vi "J1939 - SPN Indicator.vi"() -> ()   [LabVIEW 2023, in "J1939 Workspace Object.lvlib"]
doc: "Sample numeric display item."
uses:
  J1939 Workspace Object.lvlib
  <vilib>/NI VeriStand/Display Template Support/DisplayTemplateSupport.llb/cluster_Screen Item Settings.ctl
  <vilib>/NI VeriStand/Display Template Support/DisplayTemplateSupport.llb/cluster_Graph Scale Settings.ctl
  <vilib>/NI VeriStand/Display Template Support/DisplayTemplateSupport.llb/cluster_Graph Plot Settings.ctl
  NationalInstruments.VeriStand.SystemStorage
  Addon/Addon Shared/Types/SPN Properties.ctl
  <vilib>/NI VeriStand/Display Template Support/DisplayTemplateSupport.llb/enum_Display Template Handler Minimal To Workspace.ctl
  <vilib>/NI VeriStand/Display Template Support/DisplayTemplateSupport.llb/enum_Display Template Handler Minimal To Widget Msg.ctl
  <vilib>/NI VeriStand/Execution/Workspace/NI VeriStand - Get Single Channel Value.vi
  <vilib>/NI VeriStand/Display Template Support/DisplayTemplateSupport.llb/sub_Display Template Handler Custom.vi
  <vilib>/NI VeriStand/Execution/Workspace/NI_VS Workspace ExecutionAPI.lvlib
  Workspace Shared/J1939 Workspace Shared.lvlib
  Addon/Addon Shared/J1939 Addon Shared.lvlib
panel:
  out "Scale Info":T1
  in  "NIVS.System Definition Root":refnum<k24>
  out "Raw":u64 format="%.0x"
  out "MSB":u8 format="%.0x"
  in  "Item.Data":T2
  out "Numeric":dbl format="%.2f"
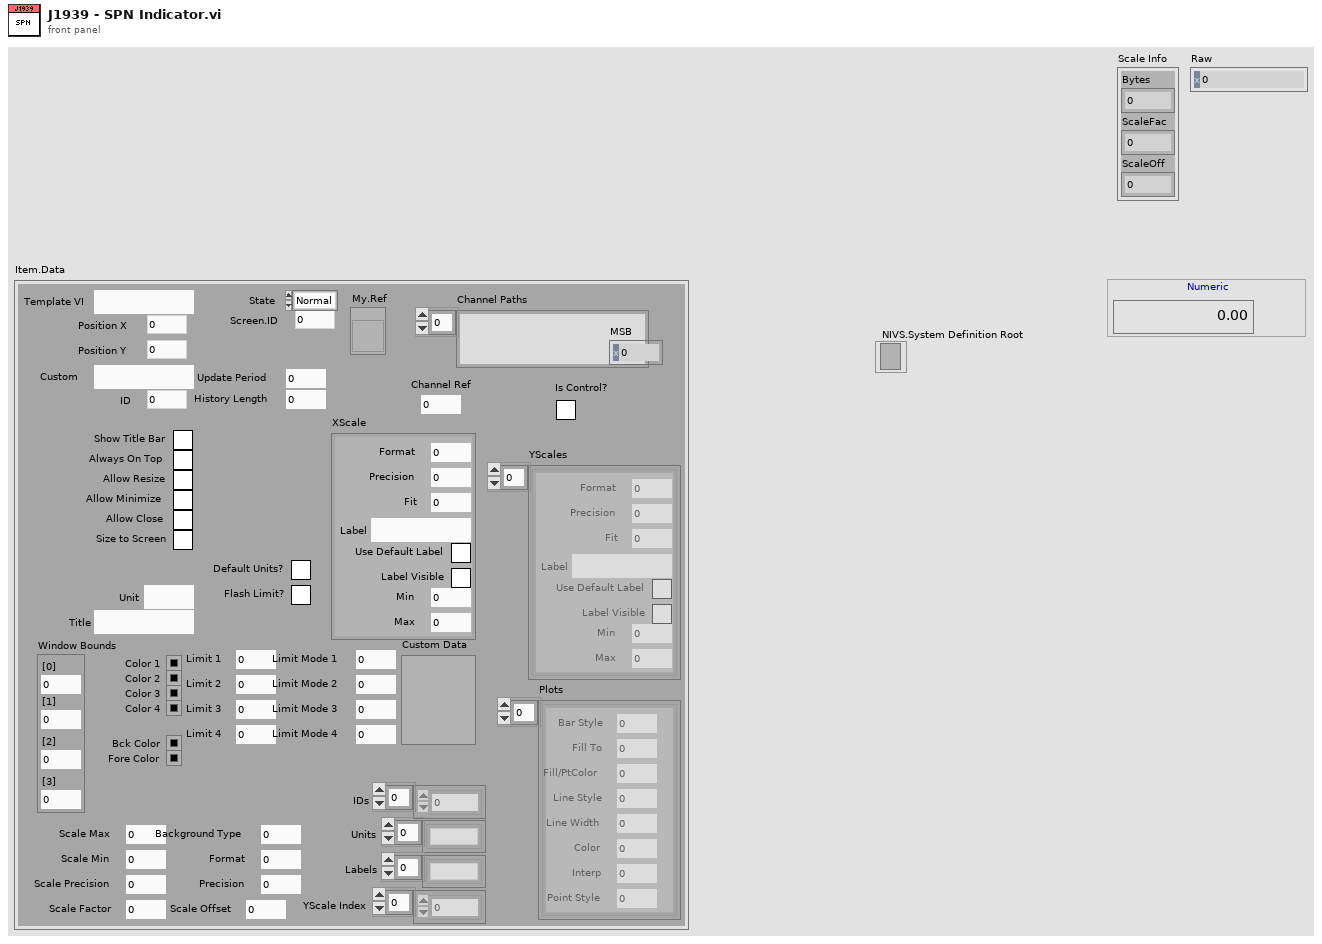
[diagram p1: front panel]
types:
  T1 = typedef "J1939 Addon Shared.lvlib/SPN Properties.ctl" = cluster{"Bytes":u32, "ScaleFac":dbl, "ScaleOff":dbl}
  T2 = typedef "cluster_Screen Item Settings.ctl" = cluster{"Template VI":string, "Position X":i32, "Position Y":i32, "Custom":string, "Show Title Bar":bool, "ID":i32, "Always On Top":bool, "Allow Resize":bool, "Allow Minimize":bool, "Allow Close":bool, "Size to Screen":bool, "Screen.ID":i32, "State":enum16{"Normal", "New"}, "Title":string, "Window Bounds":cluster{"[0]":i16, "[1]":i16, "[2]":i16, "[3]":i16}, "Channel Ref":u64, "Unit":string, "Default Units?":bool, "Flash Limit?":bool, "Color 1":u32, "Color 2":u32, "Color 3":u32, "Color 4":u32, "Bck Color":u32, "Fore Color":u32, "Limit 1":dbl, "Limit 2":dbl, "Limit 3":dbl, "Limit 4":dbl, "Limit Mode 1":i32, "Limit Mode 2":i32, "Limit Mode 3":i32, "Limit Mode 4":i32, "Scale Precision":i32, "Scale Min":dbl, "Scale Max":dbl, "Format":i32, "Precision":i32, "Background Type":i32, "IDs":i32[], "Units":string[], "Labels":string[], "Scale Factor":dbl, "Scale Offset":dbl, "YScale Index":u32[], "XScale":T3, "YScales":T3[], "Plots":T4[], "Update Period":dbl, "History Length":dbl, "My.Ref":refnum<vi>, "Is Control?":bool, "Channel Paths":string[], "Custom Data":variant}
  T3 = typedef "cluster_Graph Scale Settings.ctl" = cluster{"Format":u8, "Precision":u8, "Fit":u8, "Label":string, "Use Default Label":bool, "Label Visible":bool, "Min":dbl, "Max":dbl}
  T4 = typedef "cluster_Graph Plot Settings.ctl" = cluster{"Bar Style":u8, "Fill To":i16, "Fill/PtColor":u32, "Line Style":u8, "Line Width":u8, "Color":u32, "Interp":u8, "Point Style":u8}
  T5 = typedef "enum_Display Template Handler Minimal To Workspace.ctl" = cluster{"Operation":enum16{"SetCustomData", "DeleteItem"}, "Data":variant}
  T6 = typedef "enum_Display Template Handler Minimal To Widget Msg.ctl" = enum16{"Stop", "LaunchConfigDialog"}
  T7 = cluster{"Scale Info":T1, "NodePath":string, "Name":string}
  T8 = typedef "NI_VS Workspace ExecutionAPI.lvlib/WorkspaceAPI.ctl" = refnum<k24>
  T9 = typedef "NI_VS UI Single Node Browser.lvlib/Node Ref.ctl" = refnum<k24>
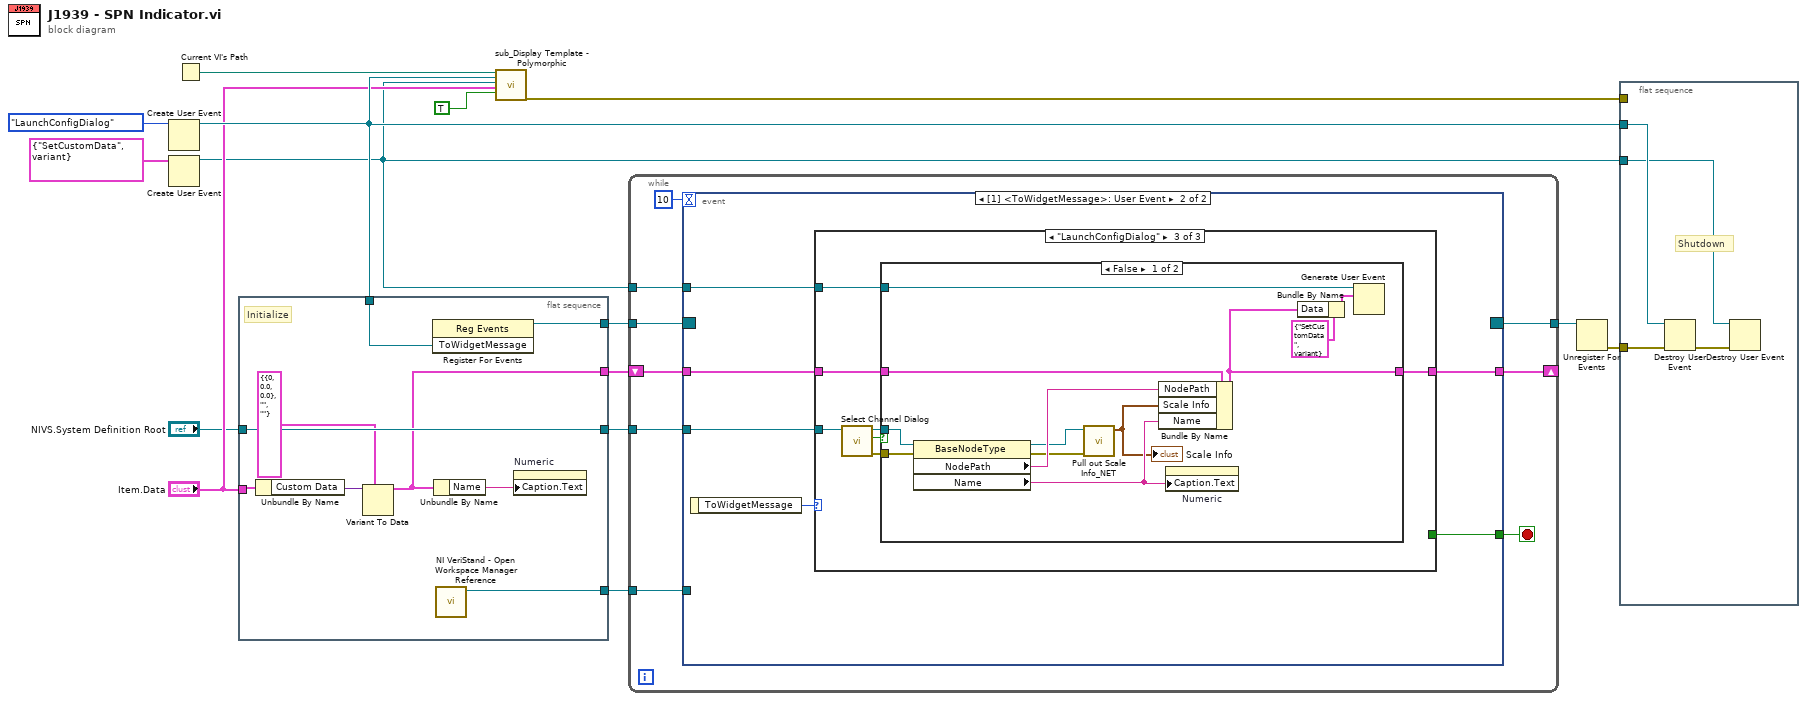
[diagram p0: block diagram]
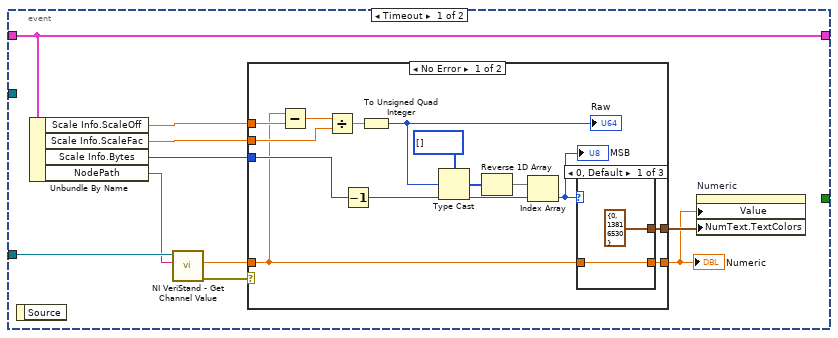
[diagram p2: hidden frame]
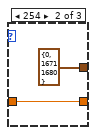
[diagram p3: hidden frame]
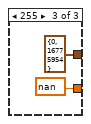
[diagram p4: hidden frame]
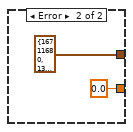
[diagram p5: hidden frame]
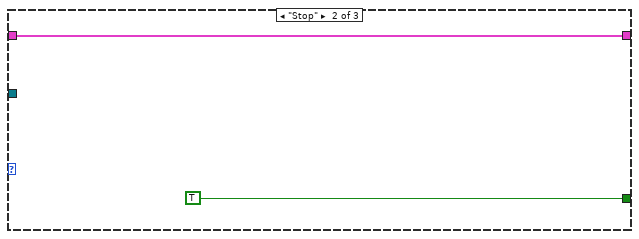
[diagram p7: hidden frame]
diagram:
  n1 = Create User Event(user event datatype=enum_Display_Template_Handler_Minimal_To_Widget_Msg."LaunchConfigDialog" ("ToWidgetMessage")) -> (user event=w12:refnum<user-event>)  [unwired: 1 in, 1 out]
  n2 = Create User Event(user event datatype=T5 {"Operation"=enum."SetCustomData", "Data"=variant} ("Data")) -> (user event=w8:refnum<user-event>)  [unwired: 1 in, 1 out]
  n3 = Current VI's Path() -> (path=w10:path)
  n4 = flat-sequence {
    tunnel: [w18] -> w13
    tunnel: w12 -> [w24]
    tunnel: "Item.Data" -> [w23]
    tunnel: [w17] -> w6
    tunnel: [w21] -> w5
    tunnel: "NIVS.System Definition Root" -> [w21]
    tunnel: [w20] -> w3
    frame #0 {
      # "Initialize"
      n5 = Unbundle By Name(w23) -> ("Custom Data"=w22:variant)
      n6 = Variant To Data(type=T7 {"Scale Info"={"Bytes"=0, "ScaleFac"=0.0, "ScaleOff"=0.0}, "NodePath"="", "Name"=""} ("Cluster"), Variant=w22) -> (data=w17:T7)  [unwired: 1 in, 1 out]
      n7 = register-events(w24) -> (reference out=w18:refnum<event-registration>)  [unwired: 2 in, 1 out]
      n8 = Unbundle By Name(w17) -> ("Name"=w16:string)
      n9 = call <vilib>:"NI VeriStand - Open Workspace Manager Reference.vi"() -> ("WorkspaceManager"=w20:T8)  [unwired: 10 in, 1 out]
      n10 = property on="Numeric" class="DigNum (strict)"("Caption.Text"=w16) -> ()  [unwired: 2 in, 2 out]
    }
  }
  n11 = call-poly <vilib>:"sub_Display Template - Polymorphic.vi"("Parent.Path"=w10, "ToWidgetEvent"=w12, "ToWorkspace"=w8, "Item.Data"="Item.Data", "Resizable"=TRUE) -> ("error out"=w15:errorcluster)  [unwired: 1 in, 13 out]
  n12 = while {
    tunnel: w13 -> [w33]
    tunnel: [w31] -> w2
    tunnel: w8 -> [w30]
    shift-right: [w28] -> _
    shift-left: w6 -> [w29]
    tunnel: w5 -> [w27]
    tunnel: w3 -> [w25]
    stop <- w32 stop-if-true
    n13 = event shown="[1] <ToWidgetMessage>: User Event" {
      selector: w33 -> [_ _]
      dyn-events: [_ _] -> w31
      timeout: 10 -> [_ _]
      tunnel: [_ w70] -> w32
      tunnel: w30 -> [_ w69]
      tunnel: w29 -> [w43 w66]
      tunnel: [w43 w68] -> w28
      tunnel: w27 -> [_ w67]
      tunnel: w25 -> [w41 _]
      event Timeout {
        n14 = event-data() -> ()  [unwired: 2 out]
        n15 = Unbundle By Name(w43) -> ("Scale Info.ScaleOff"=w42:dbl, "Scale Info.ScaleFac"=w39:dbl, "Scale Info.Bytes"=w38:u32, "NodePath"=w40:string)
        n16 = call-poly <vilib>:"NI VeriStand - Get Channel Value.vi"("Channel"=w40, "WorkspaceManager in"=w41) -> ("error out"=w34:errorcluster, "Value"=w37:dbl)  [unwired: 7 in, 1 out]
        n17 = case shown="No Error" w34 {
          tunnel: w42 -> [w57 _]
          tunnel: w39 -> [w52 _]
          tunnel: w38 -> [w51 _]
          tunnel: w37 -> [w46 _]
          tunnel: [w45 cluster{u32, u32} {16711680, 13816530} ("Cluster")] -> w36
          tunnel: [w44 0.0 ("Value")] -> w35
          frame No Error {
            n18 = Subtract(x=w46, y=w57) -> (x-y=w56:dbl)
            n19 = Divide(x=w56, y=w52) -> (x/y=w55:dbl)
            n20 = Decrement(x=w51) -> (x-1=w47:u32)
            n21 = To Unsigned Quad Integer(1:w55) -> (0:w49:u64)
            "Raw" <- w49
            n22 = Type Cast(type=u8[] [], x=w49) -> (*(type *) &x=w53:u8[])
            n23 = Reverse 1D Array(array=w53) -> (reversed array=w48:u8[])
            n24 = Index Array(array=w48, index=w47) -> (element=w50:u8)
            "MSB" <- w50
            n25 = case shown="0, Default" w50 {
              tunnel: w46 -> [w58 w61 _]
              tunnel: [w58 w61 nan] -> w44
              tunnel: [cluster{u32, u32} {0, 13816530} ("Cluster") cluster{u32, u32} {0, 16711680} cluster{u32, u32} {0, 16775954}] -> w45
              frame 0, Default {
              }
              frame 254 {
              }
              frame 255 {
              }
            }
          }
          frame Error {
          }
        }
        "Numeric" <- w35
        n26 = property on="Numeric" class="DigNum (strict)"("Value"=w35, "NumText.TextColors"=w36) -> ()  [unwired: 2 in, 2 out]
      }
      event User Event {
        n27 = event-data() -> ("ToWidgetMessage"=w71:T6)  [unwired: 1 out]
        n28 = case shown="\"LaunchConfigDialog\"" w71 {
          tunnel: [_ TRUE _] -> w70
          tunnel: w69 -> [_ _ w81]
          tunnel: w66 -> [w72 w73 w77]
          tunnel: [w72 w73 w76] -> w68
          tunnel: w67 -> [_ _ w80]
          frame Default {
          }
          frame "Stop" {
          }
          frame "LaunchConfigDialog" {
            n29 = call "Select Channel Dialog.vi"("NIVS.System Definition Root"=w80) -> ("error out"=w78:errorcluster, "Cancel?"=w75:bool, "Selected Item"=w79:T9)  [unwired: 8 in]
            n30 = case shown="False" w75 {
              tunnel: w81 -> [w93 _]
              tunnel: w79 -> [w88 _]
              tunnel: w78 -> [w87 _]
              tunnel: w77 -> [w86 w94]
              tunnel: [w85 w94] -> w76
              frame False {
                n31 = property class="BaseNodeType"(reference=w88, error in=w87) -> (reference out=w83:T9, error out=w89:errorcluster, "NodePath"=w90:string, "Name"=w84:string)
                n32 = call "Pull out Scale Info_NET.vi"("error in"=w89, "reference in"=w83) -> ("Scale Info"=w82:T1)  [unwired: 8 in, 1 out]
                "Scale Info" <- w82
                n33 = Bundle By Name(cluster=w86, "NodePath"=w90, "Scale Info"=w82, "Name"=w84) -> (w85:T7)
                n34 = property on="Numeric" class="DigNum (strict)"("Caption.Text"=w84) -> ()  [unwired: 2 in, 2 out]
                n35 = Bundle By Name(cluster=T5 {"Operation"=enum."SetCustomData", "Data"=variant} ("event data"), "Data"=w85) -> (w91:T5)
                n36 = Generate User Event(user event=w93, event data cluster=w91) -> ()  [unwired: 2 in, 2 out]
              }
              frame True {
              }
            }
          }
        }
      }
    }
  }
  n37 = Unregister For Events(event registration refnum=w2) -> (error out=w1:errorcluster)  [unwired: 1 in]
  n38 = flat-sequence {
    tunnel: w15 -> [_]
    tunnel: w1 -> [w97]
    tunnel: w12 -> [w98]
    tunnel: w8 -> [w95]
    frame #0 {
      # "Shutdown"
      n39 = Destroy User Event(user event=w98, error in=w97) -> (error out=w96:errorcluster)
      n40 = Destroy User Event(user event=w95, error in=w96) -> ()  [unwired: 1 out]
    }
  }
